vi "Load UEGO Calibration.vi"(8 "error in (no error)":errorcluster, 10 "FPGA Ref in":refnum<k20>, 11 "Device Ref in":T1 format="%.0x") -> (0 "error out":errorcluster, 1 "UEGO Present?":bool, 3 "Device Ref out":T1 format="%.0x")   [LabVIEW 2014, in "SLSC configuration Engine.lvlib"]
uses:
  SLSC configuration Engine.lvlib
  <vilib>/NI Veristand/Custom Device API/Custom Device Item Ref.ctl
  System Explorer/Type Defs/UEGO Compile Info.ctl
  Example/SPI API Test/FPGA/SLSC UEGO Calibration.ctl
  <vilib>/NI/LVFPGA Adv Session Resources/OpenByNameSubVI.vi
  Shared/Constants.vi
  <vilib>/NI Veristand/Custom Device API/Get Item Property (Variant).vi
  <vilib>/rvi/interface/common/dynamic/niFpgaEscapeDelimiterAndNull.vi
  <vilib>/Utility/error.llb/Error Cluster From Error Code.vi
  <vilib>/rvi/errors/niLvFpgaAdjustHostInterfaceError.vi
  <vilib>/FPGAPlugInAG/Dynamic/niLvFpga_Close_Dynamic.vi
  <vilib>/NI/LVFPGA Adv Session Resources/OpenByName.xnode
  <vilib>/rvi/interface/nirviReadWriteControl/nirviReadWriteControl.xnode
  <vilib>/rvi/interface/nirviCloseFPGA/nirviCloseFPGA.xnode
  <vilib>/NI Veristand/Custom Device API/Custom Device API.lvlib
  Shared/SLSC configuration Shared.lvlib
  Example/SPI API Test/FPGA/SLSC FPGA Toolkit.lvlib
  NiFpgaLv.dll
  <vilib>/rvi/interface/Simulation/niFpgaSimulationCallBeginRW.vi
  <vilib>/NI/LVFPGA Adv Session Resources/LVFPGAAdvSessionResources.lvlib
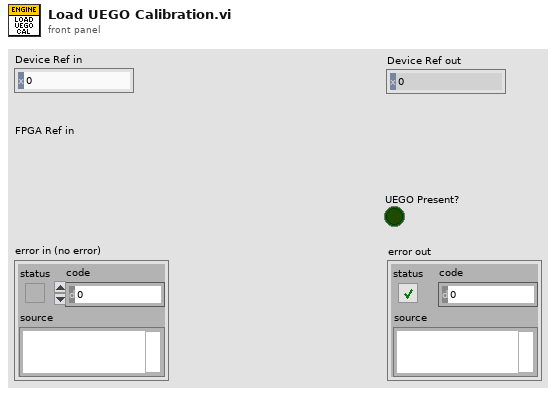
[diagram p1: front panel]
types:
  T1 = typedef "Custom Device API.lvlib/Custom Device Item Ref.ctl" = u64
  T2 = typedef "SLSC configuration Shared.lvlib/UEGO Compile Info.ctl" = cluster{"FPGA Item Name":string, "UEGOcalibration.<user name>":T3}
  T3 = typedef "SLSC FPGA Toolkit.lvlib/SLSC UEGO Calibration.ctl" = cluster{"Rack #":u8, "CS Bit Value/Slot #":u8, "Calibration Ticks":u32, "HW Settling Ticks":u32}
  T4 = cluster{"Name":string, "Depth":u32, "Write? (Deprecated:Use Implementation)":bool, "Physical Channel":u32, "Base Address":u32, "Data Width":u32, "Data Type":enum32{"Boolean", "I8", "I16", "I32", "I64", "U8", "U16", "U32", "U64", "FXP", "CustomControl", "SGL"}, "FXP Properties":variant, "Write Window Address":u32, "Implementation":enum16{"niFpgaTargetToHost", "niFpgaHostToTarget", "niFpgaPeerToPeerWriter", "niFpgaPeerToPeerReader", "niCoreTargetToHost", "niCoreHostToTarget"}, "Control Set":u32}[]
  T5 = cluster{"Name":string, "type":variant, "indicator?":bool}[]
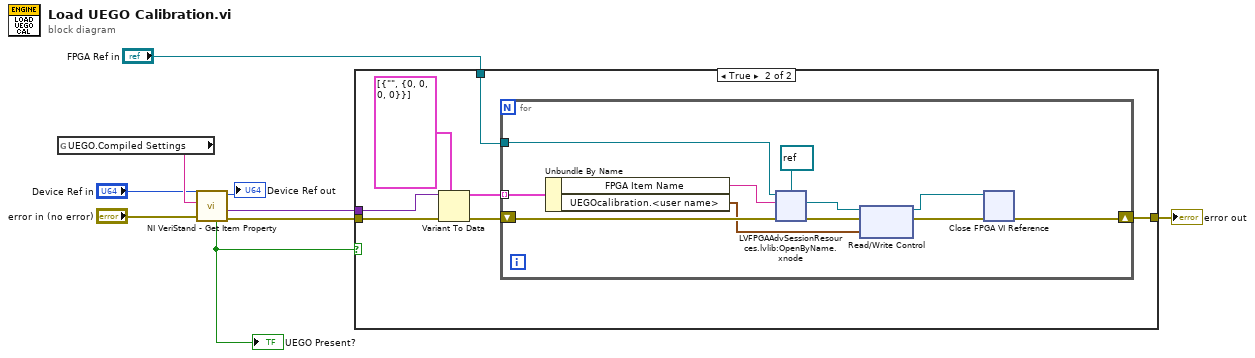
[diagram p0: block diagram]
diagram:
  n1 = global read "Constants.vi" "UEGO.Compiled Settings"() -> (w9:string)
  n2 = call-poly <vilib>:"NI VeriStand - Get Item Property.vi"("error in (no error)"="error in (no error)", "Property Name"=w9, "Item Ref in"="Device Ref in") -> ("error out"=w7:errorcluster, "Value"=w8:variant, "Item Ref out"=→"Device Ref out":T1, "Found?"=w2:bool)  [unwired: 5 in]
  "UEGO Present?" <- w2
  n3 = case shown="True" w2 {
    tunnel: w8 -> [_ w16]
    tunnel: w7 -> [w10 w15]
    tunnel: "FPGA Ref in" -> [_ w12]
    tunnel: [w10 w11] -> w3
    frame False {
    }
    frame True {
      n4 = Variant To Data(error in=w15, type=T2[] [{"FPGA Item Name"="", "UEGOcalibration.<user name>"={"Rack #"=0, "CS Bit Value/Slot #"=0, "Calibration Ticks"=0, "HW Settling Ticks"=0}}], Variant=w16) -> (data=w13:T2[], error out=w14:errorcluster)
      n5 = for {
        tunnel: w13 -> [w26] mode=indexing
        tunnel: w12 -> [w24]
        shift-right: [w18] -> w11
        shift-left: w14 -> [w28]
        n6 = Unbundle By Name(w26) -> ("FPGA Item Name"=w25:string, "UEGOcalibration.<user name>"=w21:T3)
        n7 = xnode "LVFPGAAdvSessionResources.lvlib:OpenByName.xnode"("FPGA VI Reference in"=w24, "Resource name in"=w25, "Single resource reference type in"=refnum<k20> refnum ("Single resource reference out"), "Error in"=w28) -> ("Single resource reference out"=w23:refnum<k20>, "Error out"=w22:errorcluster)  [unwired: 1 out]
        n8 = xnode "Read/Write Control"("FPGA VI Reference In"=w23, "error in"=w22, "Value"=w21) -> ("FPGA VI Reference Out"=w19:refnum<k20>, "error out"=w20:errorcluster)
        n9 = xnode "Close FPGA VI Reference"("FPGA VI Reference In"=w19, "error in"=w20) -> ("error out"=w18:errorcluster)
      }
    }
  }
  "error out" <- w3
